vi "2-1 상태머신.vi"() -> ()   [LabVIEW 2014]
uses:
  <vilib>/Analysis/NI_AALBase.lvlib
panel:
  out "웨이브폼 그래프":dbl[](graph)
  in  "정지":bool
  in  "삼각":bool
  in  "Sine":bool
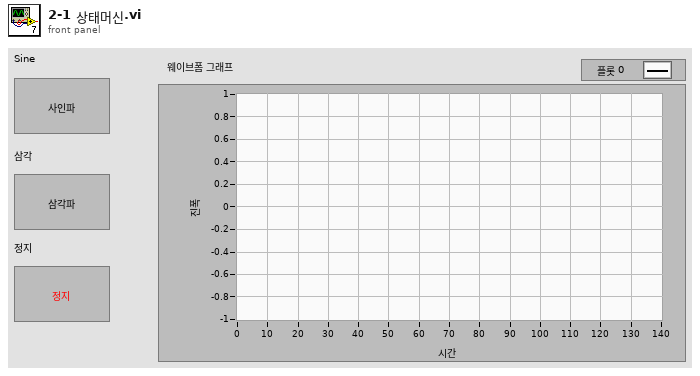
[diagram p1: front panel]
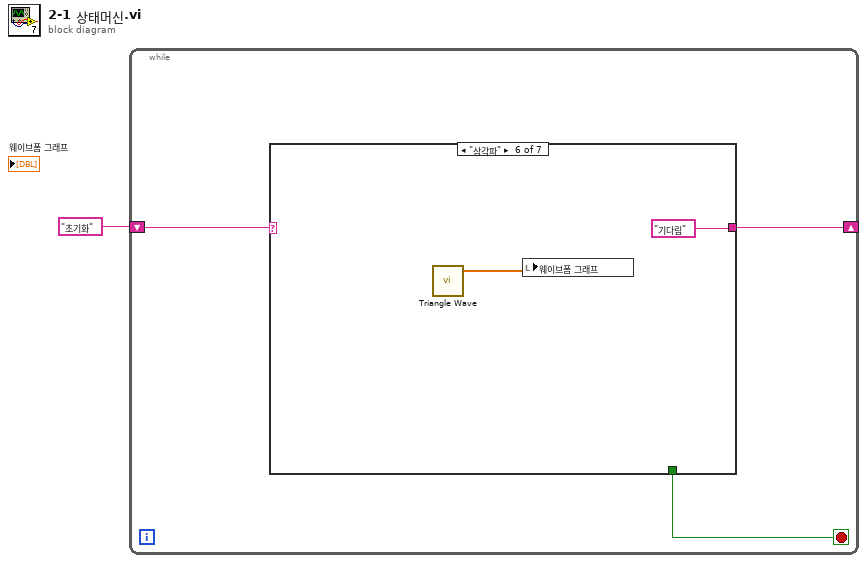
[diagram p0: block diagram]
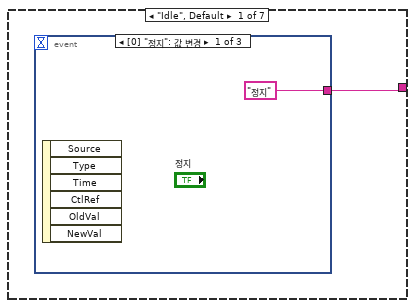
[diagram p2: hidden frame]
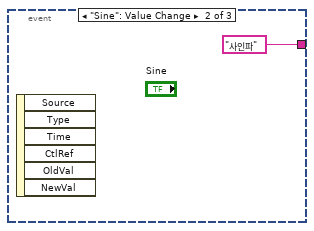
[diagram p3: hidden frame]
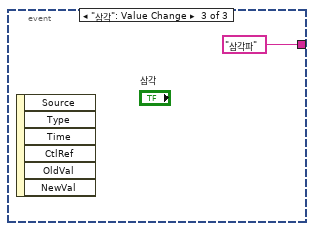
[diagram p4: hidden frame]
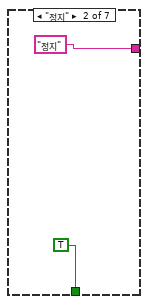
[diagram p5: hidden frame]
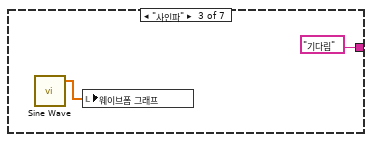
[diagram p6: hidden frame]
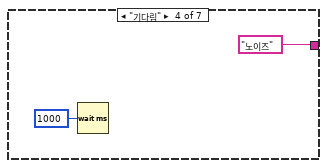
[diagram p7: hidden frame]
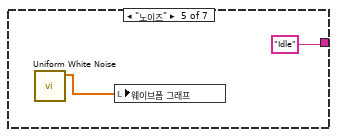
[diagram p8: hidden frame]
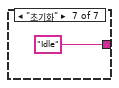
[diagram p9: hidden frame]
diagram:
  n1 = while {
    shift-right: [w3] -> _
    shift-left: "초기화" -> [w4]
    stop <- w2 stop-if-true
    n2 = case shown="\"삼각파\"" w4 {
      tunnel: [w5 "정지" "기다림" "노이즈" "Idle" "기다림" "Idle"] -> w3
      tunnel: [_ TRUE _ _ _ _ _] -> w2
      frame "Idle", Default {
        n3 = event shown="[0] \"정지\": 값 변경" {
          selector: _ -> [_ _ _]
          dyn-events: _ -> [_ _ _]
          timeout: _ -> [_ _ _]
          tunnel: ["정지" "사인파" "삼각파"] -> w5
          event "정지": Value Change {
            n4 = event-data() -> ()  [unwired: 1 in, 6 out]
          }
          event "Sine": Value Change {
            n5 = event-data() -> ()  [unwired: 1 in, 6 out]
          }
          event "삼각": Value Change {
            n6 = event-data() -> ()  [unwired: 1 in, 6 out]
          }
        }
      }
      frame "정지" {
      }
      frame "사인파" {
        n7 = call <vilib>:"Sine Wave.vi"() -> ("sine wave"=w11:dbl[])  [unwired: 5 in, 2 out]
        n8 = local write "웨이브폼 그래프"(w11) -> ()
      }
      frame "기다림" {
        n9 = Wait (ms)(milliseconds to wait=u32 1000 ("대기 시간(ms)")) -> ()  [unwired: 1 out]
      }
      frame "노이즈" {
        n10 = call <vilib>:"Uniform White Noise.vi"() -> ("uniform white noise"=w15:dbl[])  [unwired: 10 in, 1 out]
        n11 = local write "웨이브폼 그래프"(w15) -> ()
      }
      frame "삼각파" {
        n12 = call <vilib>:"Triangle Wave.vi"() -> ("triangle wave"=w18:dbl[])  [unwired: 5 in, 2 out]
        n13 = local write "웨이브폼 그래프"(w18) -> ()
      }
      frame "초기화" {
      }
    }
  }
